vi "Execute with Process Model Explicit Model.vi"() -> ()   [LabVIEW 2020]
uses:
  SequenceFile/Get Process Model.vi
  SequenceFile/Get Path.vi
  Execution/Set Entry Sequence.vi
  Execution/Set Sequence File.vi
  Execution/Set Process Model.vi
  Execution/Get Result Status.vi
  SequenceFile/SequenceFile.lvclass
  Engine/Engine.lvclass
  Execution/Execution.lvclass
panel:
  in  "Entry Point":string="Single Pass"
  out "Status":string
  in  "Model":T1(tab)
  out "File Model Name":string
  out "Station Model Name":string
  in  "Model Path":path
  in  "SequenceFile Path":path=path "C:/Users/Public/Documents/National Instruments/TestStand 2019 (32-bit)/Examples/Demos/Computer Motherboard Test/LabVIEW/Computer Motherboard Test Sequence.seq"
  # "1."
  # "2."
  # "3."
  # "4."
  # "1. Select the sequence file you'd like to run.\n\n2. Configure the process model you want to run with.\n\n3. If specifying a specific model, select the model file to run with. Otherwise the indicator will update to show the process model that will be used based on the file / station configuration.\n\n4. Enter the name of the entry point to use in the process model. This is usually 'Test UUTs' or 'Single Pass' for models that ship with TestStand."
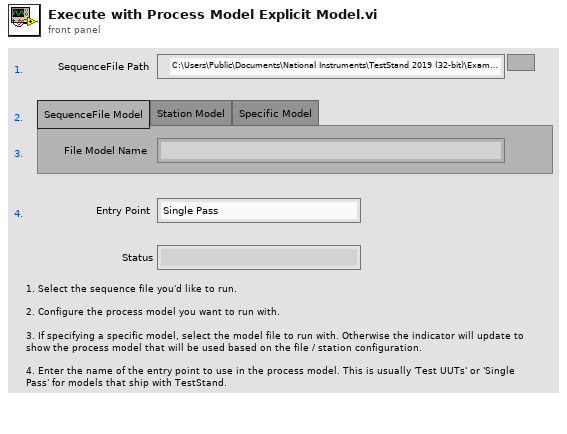
[diagram p1: front panel]
types:
  T1 = enum32{"SequenceFile Model", "Station Model", "Specific Model"}
  T2 = typedef "TSS.lvlib/Engine.lvclass/Session Handle.ctl" = refnum<data-value>
  T3 = typedef "TSS.lvlib/SequenceFile.lvclass/Session Handle.ctl" = refnum<data-value>
  T4 = typedef "TSS.lvlib/Execution.lvclass/Session Handle.ctl" = refnum<data-value>
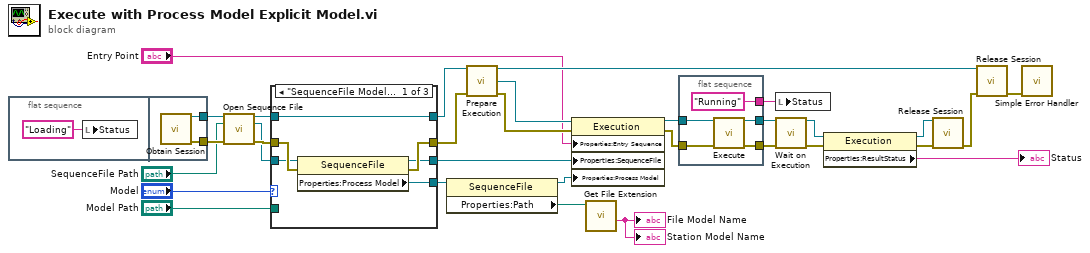
[diagram p0: block diagram]
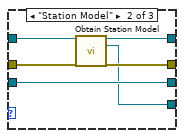
[diagram p2: hidden frame]
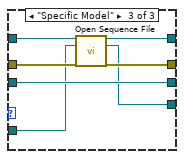
[diagram p3: hidden frame]
diagram:
  n1 = flat-sequence {
    tunnel: [w34] -> w28
    tunnel: [w33] -> w15
    frame #0 {
      n2 = local write "Status"("Loading" ("Status")) -> ()
    }
    frame #1 {
      n3 = call "Obtain Session.vi"() -> ("Session Handle"=w34:T2, "error out"=w33:errorcluster)  [unwired: 14 in]
    }
  }
  n4 = call "Open Sequence File.vi"("Engine in"=w28, "File Path"="SequenceFile Path", "error in (no error)"=w15) -> ("Session Handle out"=w27:T2, "SequenceFile"=w26:T3, "error out"=w31:errorcluster)  [unwired: 10 in]
  n5 = case shown="\"SequenceFile Model\"" "Model" {
    tunnel: "Model Path" -> [_ _ w47]
    tunnel: w27 -> [w35 w46 w52]
    tunnel: w26 -> [w38 w44 w53]
    tunnel: [w37 w41 w48] -> w25
    tunnel: [w35 w45 w51] -> w22
    tunnel: [w36 w44 w53] -> w10
    tunnel: w31 -> [w40 w43 w50]
    tunnel: [w39 w42 w49] -> w14
    frame "SequenceFile Model" {
      n6 = property class="SequenceFile"(reference=w38, error in=w40) -> (reference out=w36:T3, error out=w39:errorcluster, "Properties:Process Model"=w37:T3)
    }
    frame "Station Model" {
      n7 = call "Obtain Station Model.vi"("Session Handle in"=w46, "error in (no error)"=w43) -> ("Session Handle out"=w45:T2, "Station Model"=w41:T3, "error out"=w42:errorcluster)  [unwired: 11 in]
    }
    frame "Specific Model" {
      n8 = call "Open Sequence File.vi"("Engine in"=w52, "File Path"=w47, "error in (no error)"=w50) -> ("Session Handle out"=w51:T2, "SequenceFile"=w48:T3, "error out"=w49:errorcluster)  [unwired: 10 in]
    }
  }
  n9 = property class="SequenceFile"(reference=w25) -> (reference out=w20:T3, "Properties:Path"=w24:path)  [unwired: 1 in, 1 out]
  n10 = call "Prepare Execution.vi"("Session Handle in"=w22, "error in (no error)"=w14) -> ("Session Handle out"=w11:T2, "Execution"=w21:T4, "error out"=w13:errorcluster)  [unwired: 11 in]
  n11 = property class="Execution"(reference=w21, error in=w13, "Properties:Entry Sequence"="Entry Point", "Properties:SequenceFile"=w10, "Properties:Process Model"=w20) -> (reference out=w19:T4, error out=w16:errorcluster)
  n12 = call <vilib>:"Get File Extension.vi"("file"=w24) -> ("filename without extension"=→"File Model Name" →"Station Model Name":string)  [unwired: 6 in, 4 out]
  n13 = flat-sequence {
    tunnel: w19 -> [w58]
    tunnel: [w57] -> w18
    tunnel: [w56] -> w17
    tunnel: w16 -> [w55]
    tunnel: ["Running" ("Status")] -> w2
    frame #0 {
      n14 = call "Execute.vi"("Session Handle in"=w58, "error in (no error)"=w55) -> ("Session Handle out"=w57:T4, "error out"=w56:errorcluster)  [unwired: 12 in]
    }
  }
  n15 = local write "Status"(w2) -> ()
  n16 = call "Wait on Execution.vi"("Session Handle in"=w18, "error in (no error)"=w17) -> ("Session Handle out"=w9:T4, "error out"=w8:errorcluster)  [unwired: 11 in, 1 out]
  n17 = property class="Execution"(reference=w9, error in=w8) -> (reference out=w6:T4, error out=w7:errorcluster, "Properties:ResultStatus"=→"Status":string)
  n18 = call "Release Session.vi"("Session Handle"=w6, "error in (no error)"=w7) -> ("error out"=w12:errorcluster)  [unwired: 13 in]
  n19 = call "Release Session.vi"("Session Handle"=w11, "error in (no error)"=w12) -> ("error out"=w4:errorcluster)  [unwired: 13 in]
  n20 = call <vilib>:"Simple Error Handler.vi"("error in (no error)"=w4) -> ()  [unwired: 4 in, 5 out]
